vi "Create Channels.vi"(8 "error in (no error)":errorcluster, 10 "Channels to Create in":T1[](array[typedef]) {"Custom Config Data" format="%x"}, 11 "CIFCorePlugin in":refnum<class "CIFCorePlugin.lvclass">) -> (0 "error out":errorcluster, 2 "Channels to Create out":T1[](array[typedef]) {"Custom Config Data" format="%x"}, 3 "CIFCorePlugin out":refnum<class "CIFCorePlugin.lvclass">)   [LabVIEW 2021, in "CIFCorePlugin.lvclass"]
uses:
  CIFCorePlugin.lvclass
  Channels/ChannelRegistrar/typedef/Channel Definition.ctl
  <vilib>/CIF Foundation/CIF Channels Core/CIFChannels/Typedef/Direction.ctl
  Channels/ChannelRegistrar/typedef/Registered Channel Types.ctl
  CIFCorePlugin.lvclass/CIFCorePlugin.ctl
  <vilib>/CIF Foundation/CIF Channels Core/CIFChannels/CIFChannels.lvclass/CIFChannels.ctl
  Channels/CIFChannelMng/CIFChannelMng.lvclass/CIFChannelMng.ctl
  <vilib>/CIF Foundation/CIF Channels Core/CIPC_Channels/FIFO_U8/CIPC U8 Array FIFO.vi
  <vilib>/CIF Foundation/CIF Channels Core/CIPC_Channels/FIFO_CAN/CIPC CAN FIFO.vi
  <vilib>/CIF Foundation/CIF Channels Core/CIPC_Channels/FIFO_L2Enet/CIPC L2Enet FIFO.vi
  <vilib>/CIF Foundation/CIF Channels Core/CIPC_Channels/FIFO_DAQ/CIPC DAQ FIFO.vi
  <vilib>/CIF Foundation/CIF Channels Core/CIPC_Channels/FIFO_Universal/CIPC Universal FIFO.vi
  <vilib>/CIF Foundation/CIF Channels Core/CIFChannels/Accessors/Read Name.vi
  <vilib>/CIF Foundation/CIF Channels Core/CIFChannels/Accessors/Read Custom Config Data.vi
  <vilib>/CIF Foundation/CIF Channels Core/CIFChannels/Accessors/Read Type.vi
  <vilib>/CIF Foundation/CIF Channels Core/CIFChannels/Accessors/Read Pattern.vi
  <vilib>/CIF Foundation/CIF Channels Core/CIFChannels/Accessors/Read Direction.vi
  <vilib>/CIF Foundation/CIF Channels Core/CIFChannels/Accessors/Read Channel State.vi
  <vilib>/CIF Foundation/CIF Channels Core/ChannelCommon/Utilities/Add Error.vi
  <vilib>/CIF Foundation/CIF Utilities/Errors/Append Error Location.vi
  <vilib>/CIF Foundation/CIF Channels Core/CIPC_Channels/Double/CIF_CIPC_Chn_Double.lvclass
  C:/Program Files/National Instruments/LabVIEW 2021/vi.lib/CIF Foundation/CIF Channels Core/CIFChannels/CIFChannels.lvclass
  <vilib>/CIF Foundation/CIF Channels Core/CIPC_Channels/I64/CIF_CIPC_Chn_I64.lvclass
  <vilib>/CIF Foundation/CIF Channels Core/CIPC_Channels/U64/CIF_CIPC_Chn_U64.lvclass
  <vilib>/CIF Foundation/CIF Channels Core/CIPC_Channels/FIFO_U8/CIF_CIPC_Fifo_U8.lvclass
  <vilib>/CIF Foundation/CIF Channels Core/CIPC_Channels/FIFO_CAN/CIF_CIPC_CAN.lvclass
  <vilib>/CIF Foundation/CIF Channels Core/CIPC_Channels/FIFO_L2Enet/CIF_CIPC_L2Enet.lvclass
  <vilib>/CIF Foundation/CIF Channels Core/CIPC_Channels/FIFO_DAQ/CIF_CIPC_Fifo_DAQ.lvclass
  <vilib>/CIF Foundation/CIF Channels Core/CIPC_Channels/FIFO_Universal/CIF_CIPC_Universal.lvclass
  <vilib>/CIF Foundation/CIF Channels Core/CIPC_Channels/String/CIF_CIPC_Chn_String.lvclass
  <vilib>/CIF Foundation/CIF Channels Core/CIFChannels/CIFChannels.lvclass
  Channels/ChannelRegistrar/ChannelRegistrar.lvlib
  Common/CIFCoreCommon.lvlib
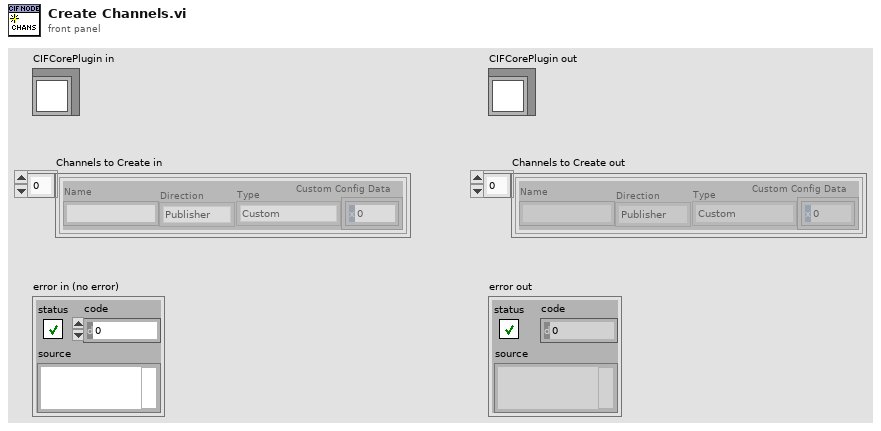
[diagram p1: front panel]
types:
  T1 = typedef "ChannelRegistrar.lvlib/Channel Definition.ctl" = cluster{"Name":string, "Direction":T2, "Type":T3, "Custom Config Data":u8[]}
  T2 = typedef "CIFChannels.lvclass/Direction.ctl" = enum16{"Publisher", "Subscriber"}
  T3 = typedef "ChannelRegistrar.lvlib/Registered Channel Types.ctl" = enum16{"Custom", "Double_Tag", "I64_Tag", "U64_Tag", "U8_FIFO", "CAN_FIFO", "L2Enet_FIFO", "DAQ_FIFO", "Universal_FIFO", "String_Tag"}
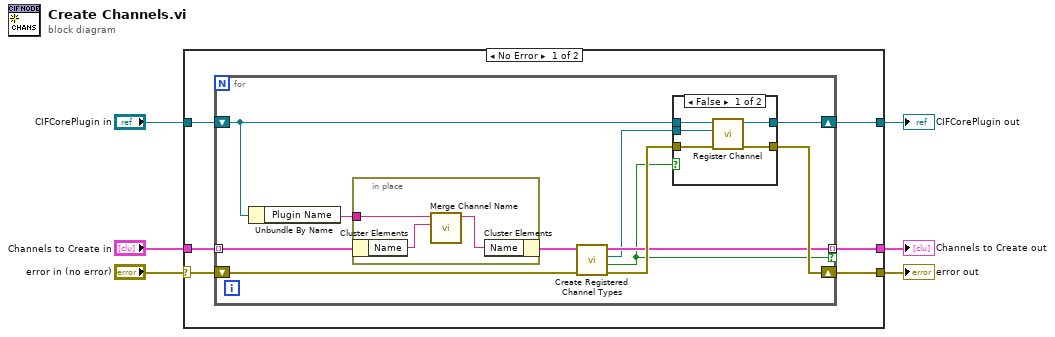
[diagram p0: block diagram]
diagram:
  n1 = case shown="No Error" "error in (no error)" {
    selector: "error in (no error)" -> [w11 w36]
    tunnel: [w9 w36] -> w1
    tunnel: [w10 w35] -> w3
    tunnel: "CIFCorePlugin in" -> [w12 w35]
    tunnel: "Channels to Create in" -> [w8 w34]
    tunnel: [w7 w34] -> w2
    frame No Error {
      n2 = for {
        tunnel: w8 -> [w16] mode=indexing
        shift-right: [w23] -> w10
        shift-left: w12 -> [w14]
        shift-right: [w21] -> w9
        shift-left: w11 -> [w22]
        tunnel: [w19] -> w7 mode=indexing if=w17
        n3 = Unbundle By Name(w14) -> ("Plugin Name"=w13:string)
        n4 = in-place {
          in-place-border: w13 -> [w26]
          n5 = in-place-cluster #1(w16) -> ("Name"=w25:string)
          n6 = call "Merge Channel Name.vi"("Child"=w25, "Parent"=w26) -> ("Channel Name"=w24:string)  [unwired: 9 in]
          n7 = in-place-cluster #1("Name"=w24) -> (w15:T1)
        }
        n8 = call "Create Registered Channel Types.vi"("error in"=w22, "Channel Definition in"=w15) -> ("error out"=w20:errorcluster, "Not Registered"=w17:bool, "Channel out"=w18:refnum<class "CIFChannels.lvclass">, "Channel Definition out"=w19:T1)  [unwired: 6 in]
        n9 = case shown="False" w17 {
          tunnel: w14 -> [w31 w33]
          tunnel: [w30 w33] -> w23
          tunnel: [w29 w32] -> w21
          tunnel: w20 -> [w28 w32]
          tunnel: w18 -> [w27 _]
          frame False {
            n10 = call "Register Channel.vi"("error in (no error)"=w28, "Channel"=w27, "CIFCorePlugin in"=w31) -> ("error out"=w29:errorcluster, "CIFCorePlugin out"=w30:refnum<class "CIFCorePlugin.lvclass">)  [unwired: 7 in]
          }
          frame True {
          }
        }
      }
    }
    frame Error {
    }
  }
  "error out" <- w1
  "CIFCorePlugin out" <- w3
  "Channels to Create out" <- w2
